vi "midi-track.get_relative_time.vi"(8 "error in (no error)":errorcluster, 10 "Track Number":i32, 11 "midi-file-events in":refnum<class "midi-file-events.lvclass">) -> (0 "error out":errorcluster, 2 "file events":refnum<class "midi-file-event.lvclass">[](array[class]), 3 "midi-file-events out":refnum<class "midi-file-events.lvclass">)   [LabVIEW 2020, in "midi-file-events.lvclass"]
uses:
  midi-file-events.lvclass
  midi-file-event/midi-file-event.lvclass
  midi-file-events.lvclass/midi-file-events.ctl
  midi-file-event/midi-file-event.lvclass/midi-file-event.ctl
  midi-file-event/Delta Tiime.get.vi
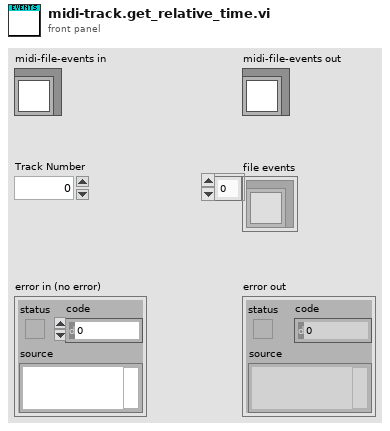
[diagram p1: front panel]
types:
  T1 = typedef "midi-file-events.lvclass/privatedata.ctl" = cluster{"ticks per quarter note (division)":i16, "Tempo Map":map{dbl, dbl}, "Track data by Track number":map{i32, map{dbl, set{refnum<class "midi-file-event.midi.lvclass">}}}}
  T2 = cluster{dbl, "element":refnum<class "midi-file-event.lvclass">}
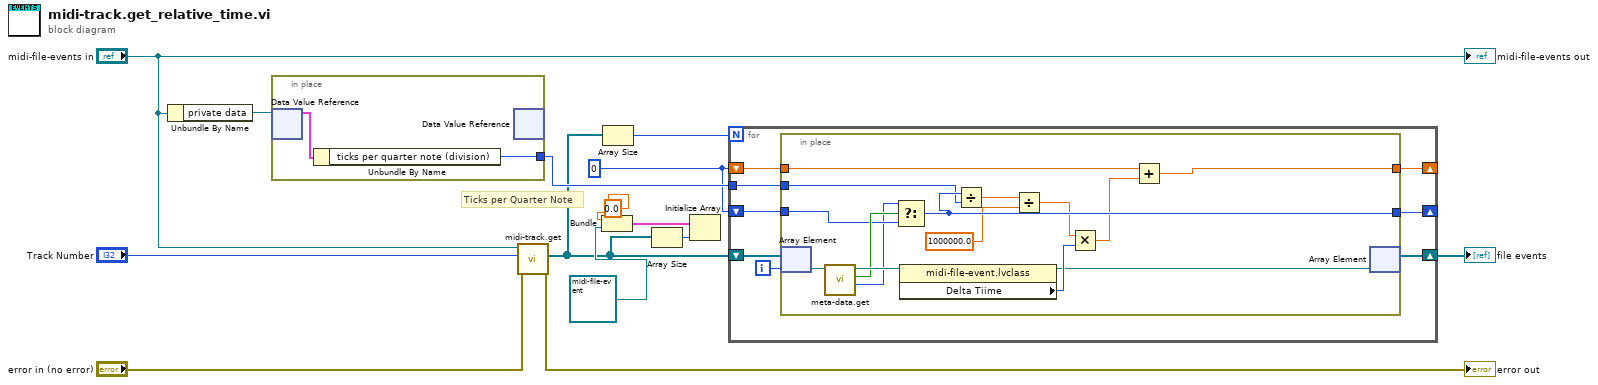
[diagram p0: block diagram]
diagram:
  w6 = u32 0 ("Delta Tiime")
  # "Ticks per Quarter Note"
  n1 = Unbundle By Name("midi-file-events in") -> ("private data"=w8:refnum<data-value>)
  n2 = in-place {
    in-place-border: [w15] -> w7
    n3 = in-place-dvr #1(w8) -> (w16:T1)  [unwired: 1 out]
    n4 = Unbundle By Name(w16) -> ("ticks per quarter note (division)"=w15:i16)
    n5 = in-place-dvr #1() -> ()  [unwired: 1 in, 2 out]
  }
  n6 = call "midi-track.get.vi"("error in (no error)"="error in (no error)", "Track Number"="Track Number", "midi-file-events in"="midi-file-events in") -> ("error out"=→"error out":errorcluster, "file events"=w2:refnum<class "midi-file-event.lvclass">[])  [unwired: 6 in, 1 out]
  n7 = Bundle(0.0, "element"=refnum<class "midi-file-event.lvclass"> refnum) -> (w3:T2)  [unwired: 1 in]
  n8 = Array Size(array=w2) -> (size(s)=w10:i32)
  n9 = Array Size(array=w2) -> (size(s)=w1:i32)
  n10 = Initialize Array(w3, w1) -> ()  [unwired: 1 out]
  n11 = for {
    N: w10 -> [_]
    shift-right: [w22] -> w14
    shift-left: w2 -> [w24]
    shift-right: [w20] -> _
    shift-left: w6 -> [w21]
    tunnel: w7 -> [w19]
    shift-right: [w18] -> _
    shift-left: w6 -> [w17]
    i -> [w23]
    n12 = in-place {
      in-place-border: w21 -> [w39]
      in-place-border: [w38] -> w20
      in-place-border: w19 -> [w31]
      in-place-border: [w32] -> w18
      in-place-border: w17 -> [w34]
      n13 = in-place-array #2(w24, w23) -> (w37:refnum<class "midi-file-event.lvclass">)
      n14 = call "meta-data.get.vi"("midi-file-event in"=w37) -> ("microseconds per quarter note"=w33:i32, "New Tempo"=w35:bool, "midi-file-event out"=w36:refnum<class "midi-file-event.lvclass">)  [unwired: 7 in, 1 out]
      n15 = Select(t=w33, s=w35, f=w34) -> (s? t:f=w32:u32)
      n16 = property class="midi-file-event.lvclass"(reference=w36) -> (reference out=w25:refnum<class "midi-file-event.lvclass">, "Delta Tiime"=w27:u32)  [unwired: 1 in, 1 out]
      n17 = Divide(x=w32, y=w31) -> (x/y=w30:dbl)
      n18 = Divide(x=w30, y=1000000.0) -> (x/y=w28:dbl)
      n19 = Multiply(x=w28, y=w27) -> (x*y=w26:dbl)
      n20 = Add(x=w39, y=w26) -> (x+y=w38:dbl)
      n21 = in-place-array #2(w25) -> (w22:refnum<class "midi-file-event.lvclass">[])  [unwired: 1 out]
    }
  }
  "file events" <- w14
  "midi-file-events out" <- "midi-file-events in"
